vi "Get Tagged Object Info.vi"(7 "Context [name]":T1=enum."name", 8 "error in (no error)":errorcluster, 11 "Carya Config in":refnum<class "Carya Config.lvclass">) -> (0 "error out":errorcluster, 1 "Context":string[](array[string]), 2 "Section names":string[](array[string]), 3 "Carya Config out":refnum<class "Carya Config.lvclass">)   [LabVIEW 2013, in "Carya Config.lvclass"]
doc: "Copyright 2018, Carya Automatisering, Wiebe Walstra."
uses:
  Carya Config.lvclass
  CConfig Object/Data.ctl
  CConfig Object/CConfig Object.lvclass
  CConfig Object/Add Results Query/Add Results Query.lvclass
  CConfig Object/Step In Query/Step In Query.lvclass
  CConfig Object/If Query/If Query.lvclass
  CConfig Object/Loop Query/Match Query/Match Query.lvclass
  CConfig Object/Loop Query/All Query/All Query.lvclass
panel:
  in  "Tagged (T)\\Untagged (F) [T]":bool=TRUE
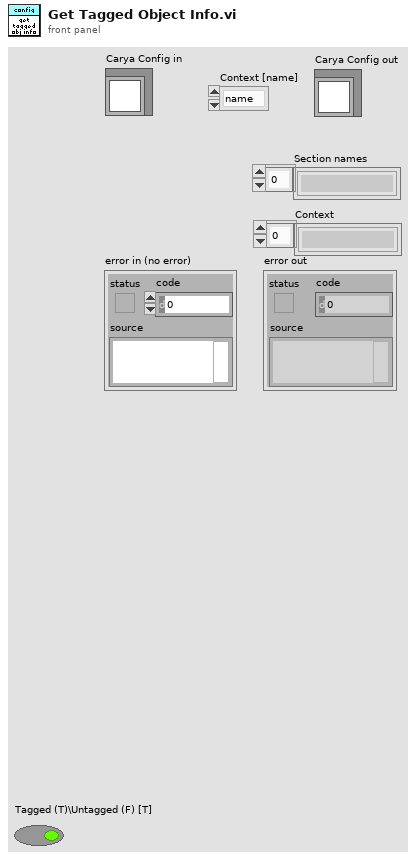
[diagram p1: front panel]
types:
  T1 = typedef "CConfig Object.lvclass/Data.ctl" = enum16{"pre", "name", "middle", "value", "post", "newline", "persistant", "tagged", "type"}
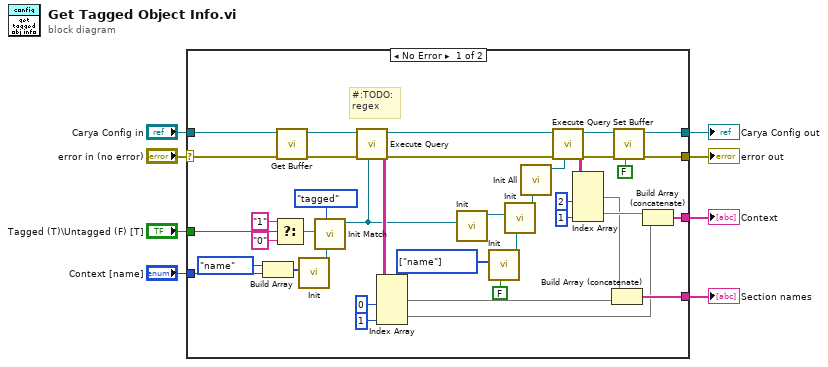
[diagram p0: block diagram]
diagram:
  n1 = case shown="No Error" "error in (no error)" {
    selector: "error in (no error)" -> [w43 w49]
    tunnel: [w45 w49] -> w5
    tunnel: [w46 w48] -> w6
    tunnel: "Carya Config in" -> [w47 w48]
    tunnel: [w14 _] -> w3
    tunnel: [w21 _] -> w2
    tunnel: "Tagged (T)\\Untagged (F) [T]" -> [w25 _]
    tunnel: "Context [name]" -> [w15 _]
    frame No Error {
      w29 = T1[] [enum."name"] items=["pre", "name", "middle", "value", "post", "newline", "persistant", "tagged", "type"] ("Data")
      # "#:TODO:\nregex"
      n2 = Build Array(Data."name" ("Data [name]"), w15) -> (w16:T1[])
      n3 = Select(t="1" ("Value"), s=w25, f="0") -> (s? t:f=w24:string)
      n4 = call-dynamic "Get Buffer.vi"("error in (no error)"=w43, "Carya Config in"=w47) -> ("error out"=w42:errorcluster, "Config"=w40:refnum<class "Carya Config.lvclass">)  [unwired: 8 in]
      n5 = call "Init.vi"("Data [name]"=w16) -> ("Find First Query out"=w23:refnum<class "Add Results Query.lvclass">)  [unwired: 9 in, 1 out]
      n6 = call "Init Match.vi"("Found"=w23, "Data [name]"=Data."tagged", "Data"=w24) -> ("Find First Query out"=w11:refnum<class "Loop Query.lvclass">)  [unwired: 7 in, 1 out]
      n7 = call-dynamic "Execute Query.vi"("Config Query in"=w11, "error in (no error)"=w42, "Carya Config in"=w40) -> ("error out"=w33:errorcluster, "Results"=w27:string[][], "Carya Config out"=w32:refnum<class "Carya Config.lvclass">)  [unwired: 4 in, 2 out]
      n8 = Index Array(array=w27, index (col) #1=0 ("index (col)"), index (col) #2=1 ("index (col)")) -> (element #1=w26:string[], element #2=w13:string[])  [unwired: 2 in]
      n9 = call "Init.vi"("Config Query"=w11) -> ("Step In Query out"=w19:refnum<class "Step In Query.lvclass">)  [unwired: 9 in, 1 out]
      n10 = call "Init.vi"("Concatenate\\Build [T, Concatenate]"=FALSE ("Concatenate\\Build [T, Concatenate]"), "Data [name]"=w29) -> ("Find First Query out"=w18:refnum<class "Add Results Query.lvclass">)  [unwired: 8 in, 1 out]
      n11 = call "Init.vi"("True"=w18, "If"=w19) -> ("Find First Query out"=w20:refnum<class "If Query.lvclass">)  [unwired: 8 in, 1 out]
      n12 = call "Init All.vi"("Found"=w20) -> ("Find First Query out"=w10:refnum<class "All Query.lvclass">)  [unwired: 9 in, 1 out]
      n13 = call-dynamic "Execute Query.vi"("Config Query in"=w10, "error in (no error)"=w33, "Carya Config in"=w32) -> ("error out"=w44:errorcluster, "Results"=w36:string[][], "Carya Config out"=w39:refnum<class "Carya Config.lvclass">)  [unwired: 4 in, 2 out]
      n14 = Index Array(array=w36, index (col) #1=2 ("disabled index (col)"), index (col) #2=1 ("index (col)")) -> (element #1=w22:string[], element #2=w41:string[])  [unwired: 2 in]
      n15 = Build Array (concatenate)(w22, w26) -> (w21:string[])
      n16 = call-dynamic "Set Buffer.vi"("Set? [T]"=FALSE, "error in (no error)"=w44, "Carya Config"=w39) -> ("error out"=w45:errorcluster, "Carya Config out"=w46:refnum<class "Carya Config.lvclass">)  [unwired: 7 in]
      n17 = Build Array (concatenate)(w41, w13) -> (w14:string[])
    }
    frame Error {
    }
  }
  "error out" <- w5
  "Carya Config out" <- w6
  "Section names" <- w2
  "Context" <- w3
